vi "load_xml.vi"(8 "error in":errorcluster, 10 "child node in":refnum<k20>, 11 "DDS.lvclass (in)":refnum<class "DDS.lvclass">) -> (0 "error out":errorcluster, 2 "child node out":refnum<k20>, 3 "DDS.lvclass":refnum<class "DDS.lvclass">)   [LabVIEW 2014, in "DDS.lvclass"]
doc: "This .vi creates a DDS settings cluster from xml.\n\nExpected format:\n\n<DDS>\n<EnableDDS>%b</EnableDDS>\n<ArrayOfDDSBoxes>\n\n<box>\n<Enable>%b</Enable>\n<DDSBoxDeviceReference.Resource>%s</DDSBoxDeviceReference.Resource>\n<DDSBoxDeviceReference.DIOPort>%u</DDSBoxDeviceReference.DIOPort>\n<DDSBoxDeviceReference.SerialClockRate units=\"kHz\">%u</DDSBoxDeviceReference.SerialClockRate>\n<ArrayOfDDSChannels>\n\n<channel>\n<Power>%b</Power>\n<ChannelParameters.RefClockRate units=\"kHz\">%f</ChannelParameters.RefClockRate>\n<ChannelParameters.FullScaleOutputPower units=\"dBm\">%f</ChannelParameters.FullScaleOutputPower>\n<RAMEnable>%b</RAMEnable>\n<RAMDestType>%u</RAMDestType>\n<RAMDefault.Frequency units=\"MHz\">%s</RAMDefault.Frequency>\n<RAMDefault.Amplitude units=\"dBm\">%s</RAMDefault.Amplitude>\n<RAMDefault.Phase units=\"rad\">%s</RAMDefault.Phase>\n<ArrayOfDDSProfiles>\n\n<profile>\n<SingleTone.Frequency units=\"MHz\">%s</SingleTone.Frequency>\n<SingleTone.Amplitude units=\"dBm\">%s</SingleTone.Amplitude>\n<SingleTone.Phase units=\"rad\">%s</SingleTone.Phase>\n<RAMMode>%u</RAMMode>\n<ZeroCrossing>%b</ZeroCrossing>\n<NoDwellHigh>%b</NoDwellHigh>\n<FunctionOrStatic>%b</FunctionOrStatic>\n<RAMFunctionSettings>%s</RAMFunctionSettings>\n<RAMStaticArray>%s</RAMStaticArray>\n</profile>\n\n</ArrayOfDDSProfiles>\n</channel>\n\n</ArrayOfDDSChannels>\n</box>\n\n</ArrayOfDDSBoxes>\n</DDS>\n\nMTL 2012 Dec 31"
uses:
  DDS.lvclass
  <resource>/objmgr/DOMUserDefRef.rc
  <vilib>/xml/NI_XML.lvlib
  <vilib>/xml/Close Reference(Node).vi
  Globals.vi
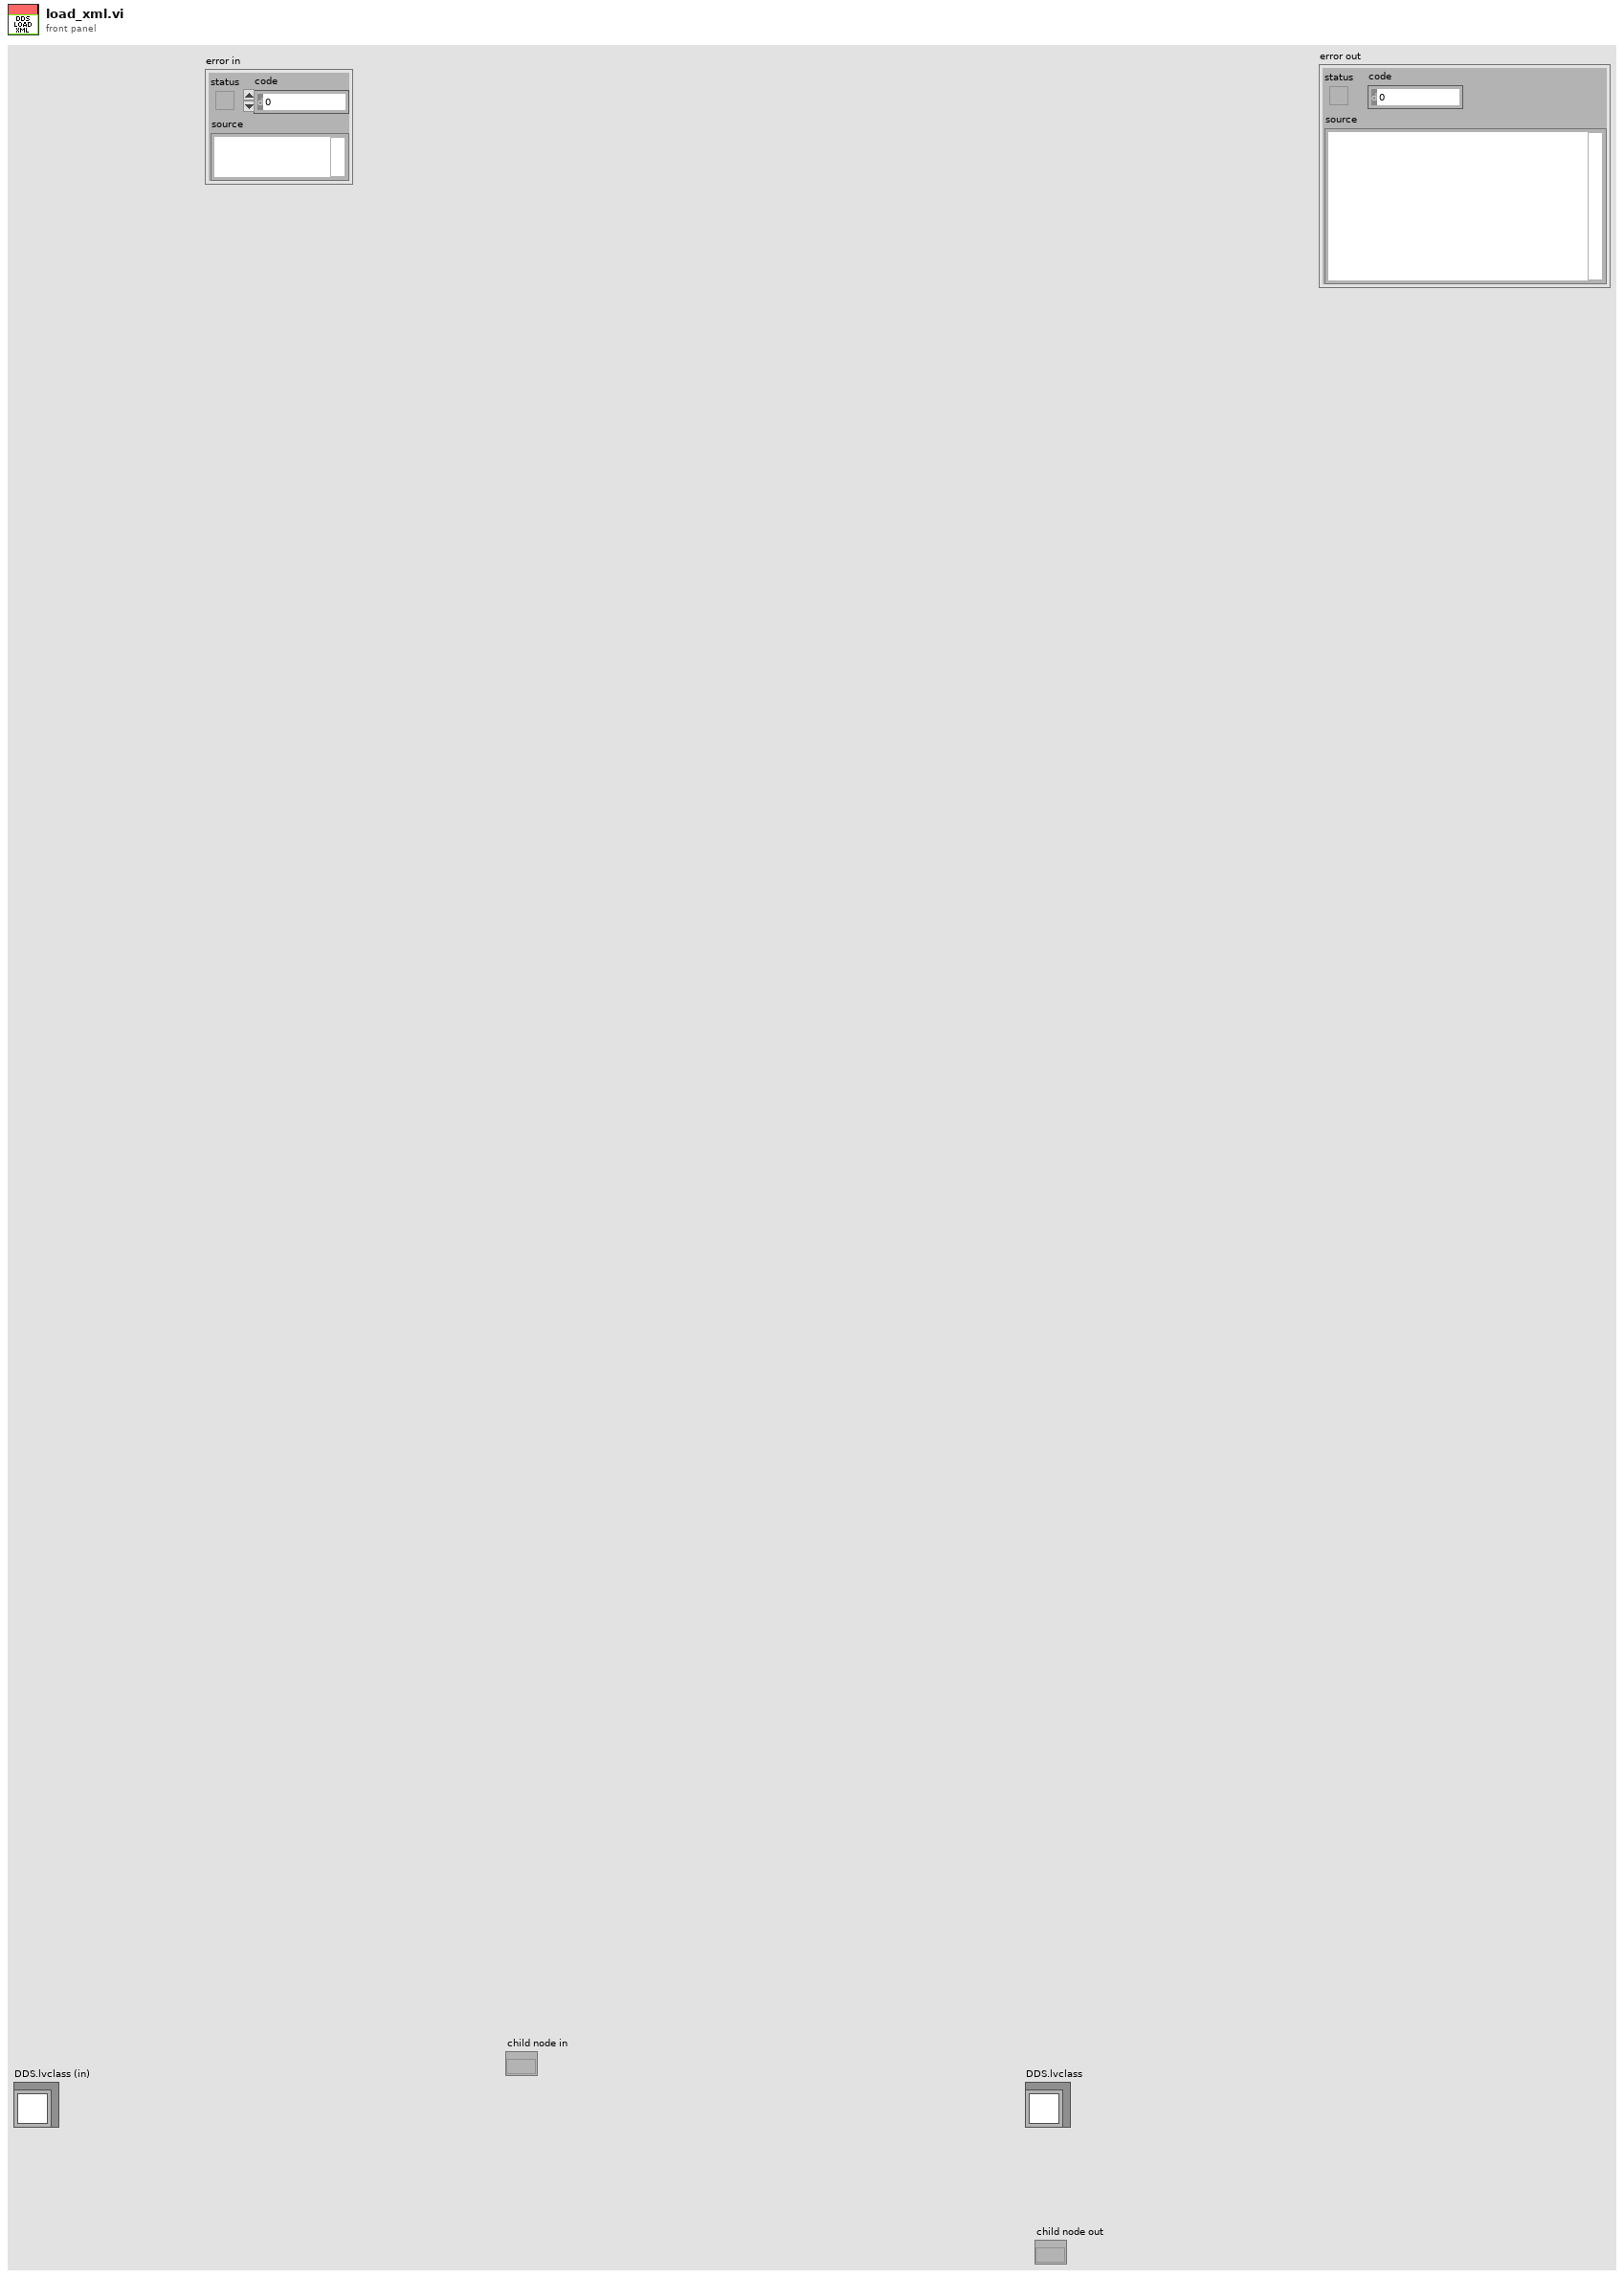
[diagram p1: front panel]
types:
  T1 = typedef "DDS.lvclass/DDS_Settings_Cluster.ctl" = cluster{"Enable DDS":bool, "Array of DDS Boxes":T2}
  T2 = typedef "DDS.lvlib/DDS Box Array.ctl" = T3[]
  T3 = typedef "DDS.lvlib/DDS Box Cluster.ctl" = cluster{"DDS box device reference":T4, "Array of DDS Channels (4)":T6, "Enable":bool, "Description":string}
  T4 = typedef "DDS.lvlib/DDS Box Device Reference.ctl" = cluster{"NI USB-8451 device reference":T5, "DIO port":u8, "Serial Clock Rate [kHz]":u16}
  T5 = typedef "ni845xControl.ctl" = refnum<k21>
  T6 = typedef "DDS.lvlib/DDS Channel Array.ctl" = T7[]
  T7 = typedef "DDS.lvlib/DDS Channel.ctl" = cluster{"Power":bool, "Channel Parameters":T8, "RAM Enable":bool, "RAM Dest Type":T9, "RAM Default":cluster{"Frequency [MHz]":string, "Amplitude [dBm]":string, "Phase Offset [rad]":string}, "Array of DDS Profiles (8)":T10, "Description":string}
  T8 = typedef "DDS.lvlib/DDS Channel Parameters.ctl" = cluster{"Ref Clock Rate [MHz]":dbl, "Full Scale Output\nPower [dBm]":dbl}
  T9 = typedef "DDS.lvlib/DDS RAM Destination.ctl" = enum16{"Frequency", "Phase", "Amplitude", "Polar"}
  T10 = typedef "DDS.lvlib/DDS Profile Array.ctl" = T11[]
  T11 = typedef "DDS.lvlib/DDS Profile.ctl" = cluster{"Single Tone":cluster{"Frequency [MHz]":string, "Amplitude [dBm]":string, "Phase Offset [rad]":string}, "RAM Mode ":T12, "Zero-crossing":bool, "No Dwell High":bool, "Function/Static":bool, "RAM Function Settings":string[], "RAM Static Array":dbl[][], "Description":string, "Time Step (us)":T13}
  T12 = typedef "DDS.lvlib/DDS RAM mode.ctl" = enum16{"Direct Switch", "Ramp Up", "Bidirectional Ramp", "Continuous Bidirectional Ramp", "Continuous Recirculate", "Direct Switch 2", "Direct Switch 3", "Direct Switch 4"}
  T13 = typedef "DDS.lvlib/DDS RAM Timestep.ctl" = dbl
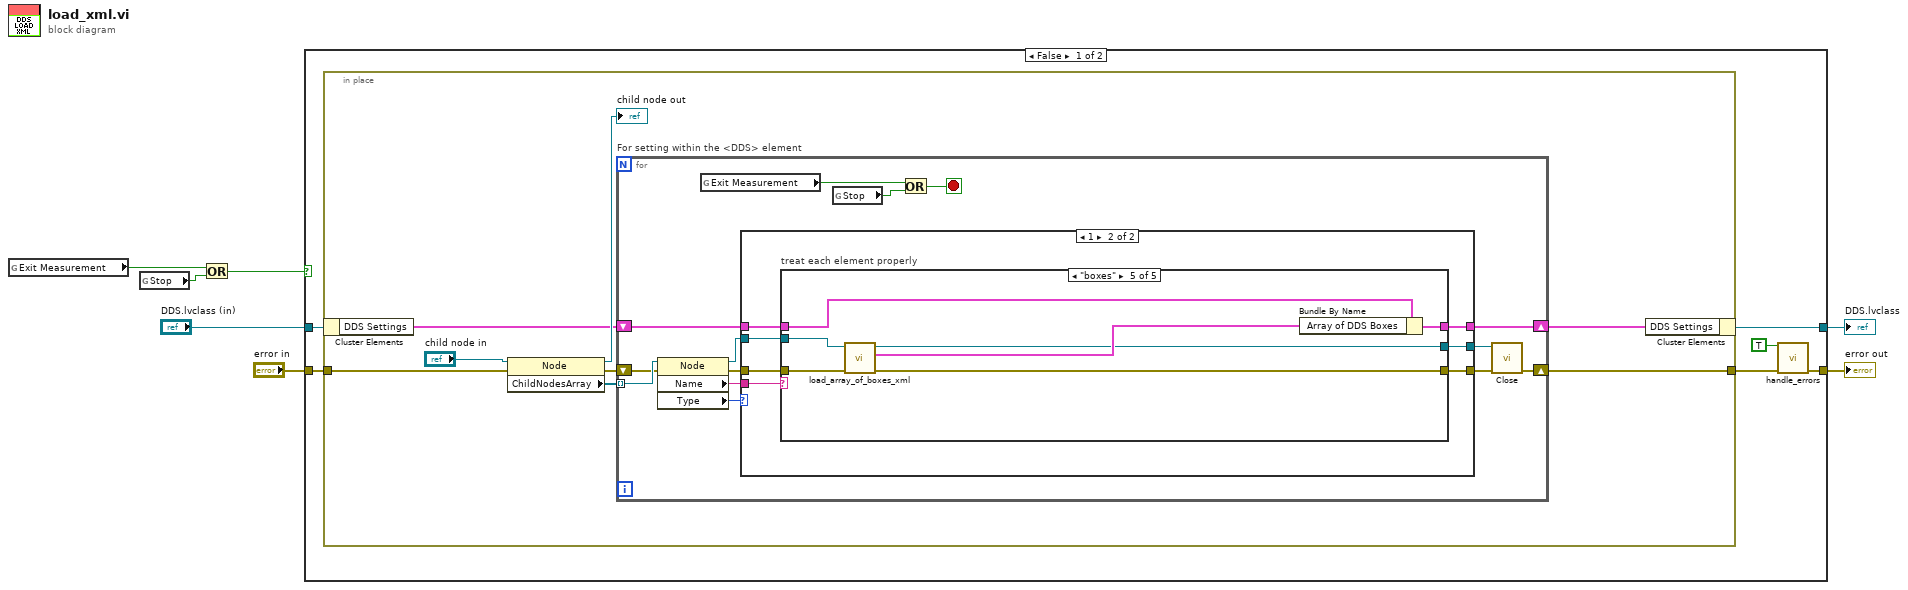
[diagram p0: block diagram]
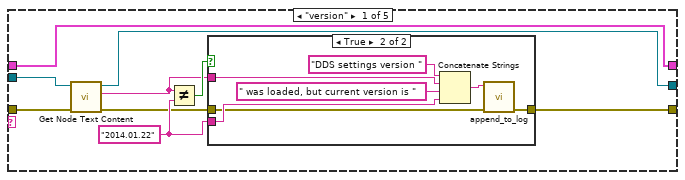
[diagram p3: hidden frame]
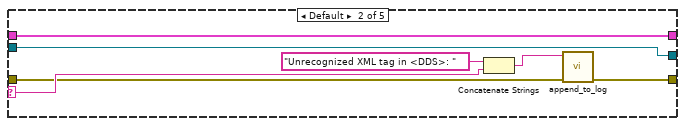
[diagram p5: hidden frame]
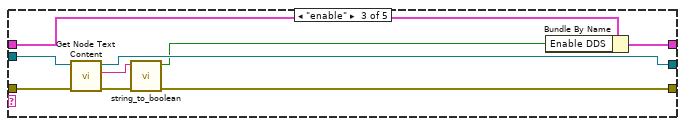
[diagram p6: hidden frame]
diagram:
  n1 = global read "Globals.vi" "Exit Measurement"() -> (w4:bool)
  n2 = global read "Globals.vi" "Stop"() -> (w3:bool)
  n3 = Or(x=w4, y=w3) -> (x .or. y?=w2:bool)
  n4 = case shown="False" w2 {
    tunnel: "DDS.lvclass (in)" -> [w13 w90]
    tunnel: [w12 w89] -> w6
    tunnel: [w9 w90] -> w5
    tunnel: "error in" -> [w8 w89]
    frame False {
      n5 = in-place {
        in-place-border: [w15] -> w11
        in-place-border: w8 -> [w14]
        n6 = in-place-cluster #1(w13) -> ("DDS Settings"=w17:T1)
        n7 = property class="Node"(reference="child node in", error in=w14) -> (reference out=→"child node out":refnum<k20>, error out=w19:errorcluster, "ChildNodesArray"=w21:refnum<k20>[])
        n8 = for "For setting within the <DDS> element" {
          tunnel: w21 -> [w27] mode=indexing
          shift-right: [w32] -> w16
          shift-left: w17 -> [w33]
          shift-right: [w29] -> w15
          shift-left: w19 -> [w26]
          stop <- w22 stop-if-true
          n9 = property class="Node"(reference=w27, error in=w26) -> (reference out=w34:refnum<k20>, error out=w30:errorcluster, "Name"=w35:string, "Type"=w25:i32)
          n10 = global read "Globals.vi" "Exit Measurement"() -> (w24:bool)
          n11 = case shown="1" w25 {
            tunnel: w35 -> [_ w45]
            tunnel: w34 -> [w37 w44]
            tunnel: w33 -> [w38 w43]
            tunnel: [w38 w42] -> w32
            tunnel: [w37 w41] -> w31
            tunnel: w30 -> [w36 w40]
            tunnel: [w36 w39] -> w28
            frame 0, Default {
            }
            frame 1 {
              n12 = case "treat each element properly" shown="\"boxes\"" w45 {
                selector: w45 -> [_ w65 _ _ _]
                tunnel: w44 -> [w46 w68 w77 w80 w82]
                tunnel: w43 -> [w48 w69 w75 w81 w87]
                tunnel: [w48 w69 w74 w81 w88] -> w42
                tunnel: [w49 w68 w78 w80 w83] -> w41
                tunnel: w40 -> [w47 w64 w76 w79 w85]
                tunnel: [w50 w63 w71 w79 w86] -> w39
                frame "version" {
                  w52 = "2014.01.22" ("y")
                  n13 = call <vilib>:"Get Node Text Content.vi"("error in (no error)"=w47, "node in"=w46) -> ("error out"=w51:errorcluster, "node text"=w53:string, "node out"=w49:refnum<k20>)  [unwired: 7 in]
                  n14 = Not Equal?(x=w53, y=w52) -> (x != y?=w54:bool)
                  n15 = case shown="True" w54 {
                    tunnel: w53 -> [_ w61]
                    tunnel: w52 -> [_ w59]
                    tunnel: w51 -> [w55 w57]
                    tunnel: [w55 w56] -> w50
                    frame False {
                    }
                    frame True {
                      n16 = Concatenate Strings("DDS settings version " ("string"), w61, " was loaded, but current version is " ("string"), w59) -> (w58:string)
                      n17 = call "append_to_log.vi"("error in"=w57, "string"=w58) -> ("error out"=w56:errorcluster)  [unwired: 9 in]
                    }
                  }
                }
                frame Default {
                  n18 = Concatenate Strings("Unrecognized XML tag in <DDS>: " ("string"), w65) -> (w66:string)
                  n19 = call "append_to_log.vi"("error in"=w64, "string"=w66) -> ("error out"=w63:errorcluster)  [unwired: 9 in]
                }
                frame "enable" {
                  n20 = call <vilib>:"Get Node Text Content.vi"("error in (no error)"=w76, "node in"=w77) -> ("error out"=w72:errorcluster, "node text"=w73:string, "node out"=w78:refnum<k20>)  [unwired: 7 in]
                  n21 = call "string_to_boolean.vi"("error in"=w72, "string"=w73) -> ("error out"=w71:errorcluster, "boolean"=w70:bool)  [unwired: 8 in]
                  n22 = Bundle By Name(cluster=w75, "Enable DDS"=w70) -> (w74:T1)
                }
                frame "description" {
                }
                frame "boxes" {
                  n23 = call "load_array_of_boxes_xml.vi"("error in"=w85, "node in"=w82) -> ("error out"=w86:errorcluster, "ArrayOfDDSBoxes"=w84:T3[], "node"=w83:refnum<k20>)  [unwired: 7 in]
                  n24 = Bundle By Name(cluster=w87, "Array of DDS Boxes"=w84) -> (w88:T1)
                }
              }
            }
          }
          n25 = global read "Globals.vi" "Stop"() -> (w23:bool)
          n26 = Or(x=w24, y=w23) -> (x .or. y?=w22:bool)
          n27 = call-poly <vilib>:"Close.vi"("error in (no error)"=w28, "node"=w31) -> ("error out"=w29:errorcluster)  [unwired: 7 in]
        }
        n28 = in-place-cluster #1("DDS Settings"=w16) -> (w9:refnum<class "DDS.lvclass">)
      }
      n29 = call "handle_errors.vi"("Exit Operation"=TRUE ("Exit Measurement"), "error in (no error)"=w11) -> ("error out"=w12:errorcluster)  [unwired: 13 in]
    }
    frame True {
    }
  }
  "error out" <- w6
  "DDS.lvclass" <- w5
